vi "Finalize.vi"(8 "error in":errorcluster, 11 "Ballard ARINC-429 Tx Scheduled Labels Execution Unit in":refnum<class "Tx Scheduled Labels Execution Unit.lvclass">) -> (0 "error out":errorcluster, 3 "Ballard ARINC-429 Tx Scheduled Labels Execution Unit out":refnum<class "Tx Scheduled Labels Execution Unit.lvclass">)   [LabVIEW 2020, in "Ballard ARINC 429 Engine.lvlib" / "Implementation.lvlib" / "Tx Scheduled Labels Execution Unit.lvclass"]
uses:
  Tx Scheduled Labels Execution Unit.lvclass
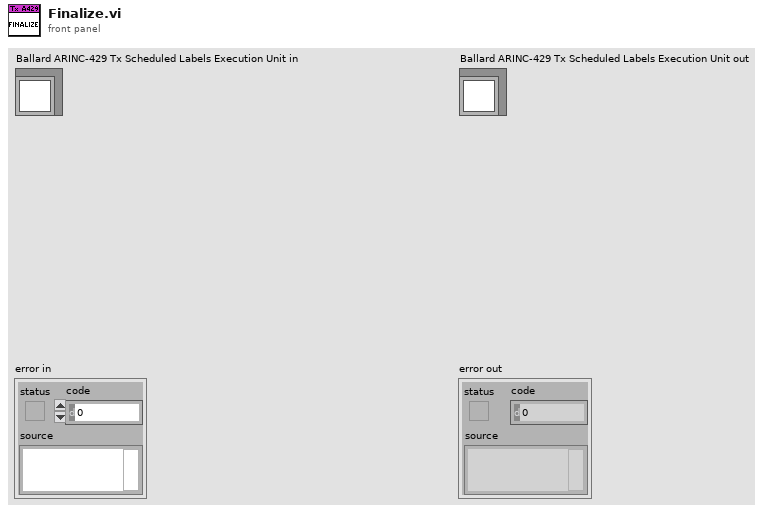
[diagram p1: front panel]
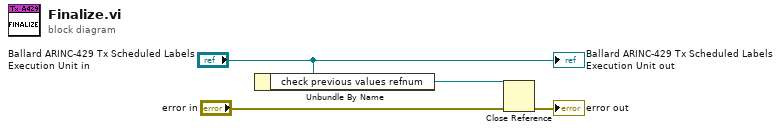
[diagram p0: block diagram]
diagram:
  n1 = Unbundle By Name("Ballard ARINC-429 Tx Scheduled Labels Execution Unit in") -> ("check previous values refnum"=w1:refnum<vi>)
  n2 = Close Reference(reference=w1, error in (no error)="error in") -> (error out=→"error out":errorcluster)
  "Ballard ARINC-429 Tx Scheduled Labels Execution Unit out" <- "Ballard ARINC-429 Tx Scheduled Labels Execution Unit in"
